vi "Cal Week.vi"(5 "time":T1) -> (2 "week":u16)   [LabVIEW 2020]
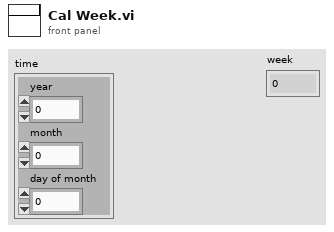
[diagram p1: front panel]
types:
  T1 = cluster{"year":u16, "month":u16, "day of month":u16}
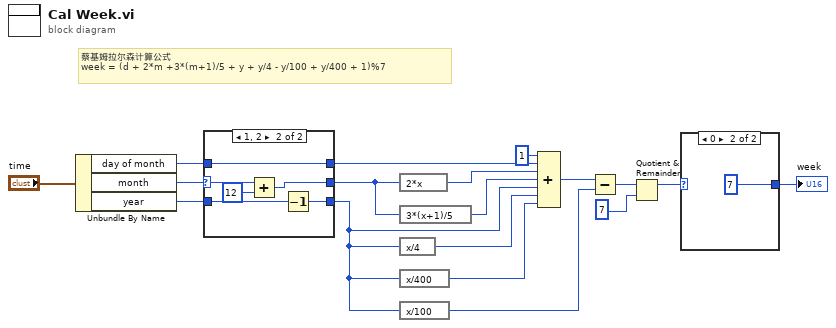
[diagram p0: block diagram]
diagram:
  # "蔡基姆拉尔森计算公式\nweek = (d + 2*m +3*(m+1)/5 + y + y/4 - y/100 + y/400 + 1)%7"
  n1 = Unbundle By Name("time") -> ("day of month"=w8:u16, "month"=w7:u16, "year"=w6:u16)
  n2 = case shown="1, 2" w7 {
    selector: w7 -> [w20 w24]
    tunnel: w8 -> [w21 w25]
    tunnel: w6 -> [w19 w27]
    tunnel: [w21 w25] -> w5
    tunnel: [w20 w23] -> w4
    tunnel: [w19 w26] -> w3
    frame Default {
    }
    frame 1, 2 {
      n3 = Add(x=w24, y=u16 12) -> (x+y=w23:u16)
      n4 = Decrement(x=w27) -> (x-1=w26:u16)
    }
  }
  n5 = expression code="2*x"(w4) -> (w17:u16)
  n6 = expression code="3*(x+1)/5"(w4) -> (w16:u16)
  n7 = expression code="x/4"(w3) -> (w15:u16)
  n8 = expression code="x/400"(w3) -> (w14:u16)
  n9 = expression code="x/100"(w3) -> (w12:u16)
  n10 = Compound Arithmetic op=ADD(u16 1 ("value"), w5, w17, w16, w3, w15, w14) -> (w13:u16)
  n11 = Subtract(x=w13, y=w12) -> (x-y=w11:u16)
  n12 = Quotient & Remainder(x=w11, y=u16 7) -> (x-y*floor(x/y)=w2:u16)  [unwired: 1 out]
  n13 = case shown="0" w2 {
    selector: w2 -> [w28 _]
    tunnel: [w28 u16 7] -> w1
    frame Default {
    }
    frame 0 {
    }
  }
  "week" <- w1
